vi "Dummy.vi"() -> ()   [LabVIEW 2020]
uses:
  Global 1.vi
panel:
  out "Report Array Header":string[](array[string])
  out "Date (DD/MM/YYYY)":string
  out "SHORT Compensation":string
  out "OPEN Compensation":string
  in  "Calibration Short : Started":bool
  in  "Open Calibration : Started":bool
  in  "Stop Button 2":bool
  out "Current LCR Voltage 2":dbl
  in  "Start Test":bool
  out "Multiplier 2":dbl format="%#_3g"
  out "Test Level value 2":dbl
  in  "Test Comments":string
  in  "Lot Date":timestamp=timestamp(3376684800 s since 1904-01-01) format="%<%x>T"
  in  "Lot Number":string
  in  "Part Number":string
  in  "Request Number":string
  out "TestSigLevel : current time":timestamp
  out "error Mult True":errorcluster
  out "error Mult False":errorcluster
  in  "TestSigLevel : Started":bool
  out "Signal Level : Elapsed time (seconds)":dbl
  in  "OK Button":bool
  in  "Stop Button":bool
  out "Current LCR Voltage":dbl
  out "Multiplier":dbl format="%#_3g"
  out "Test Level Equal":bool
  out "Test Level value":dbl
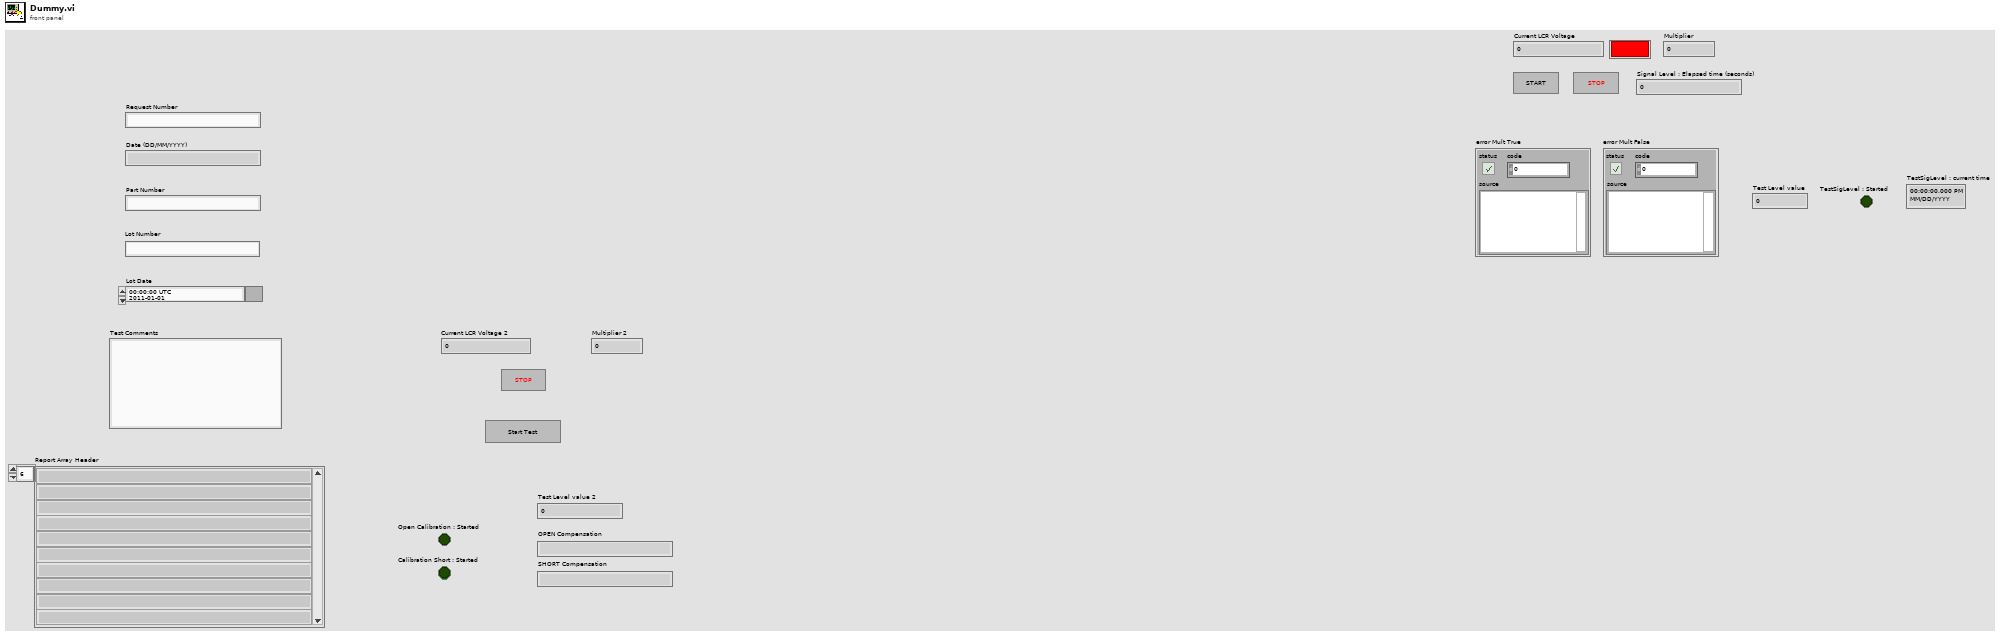
[diagram p1: front panel]
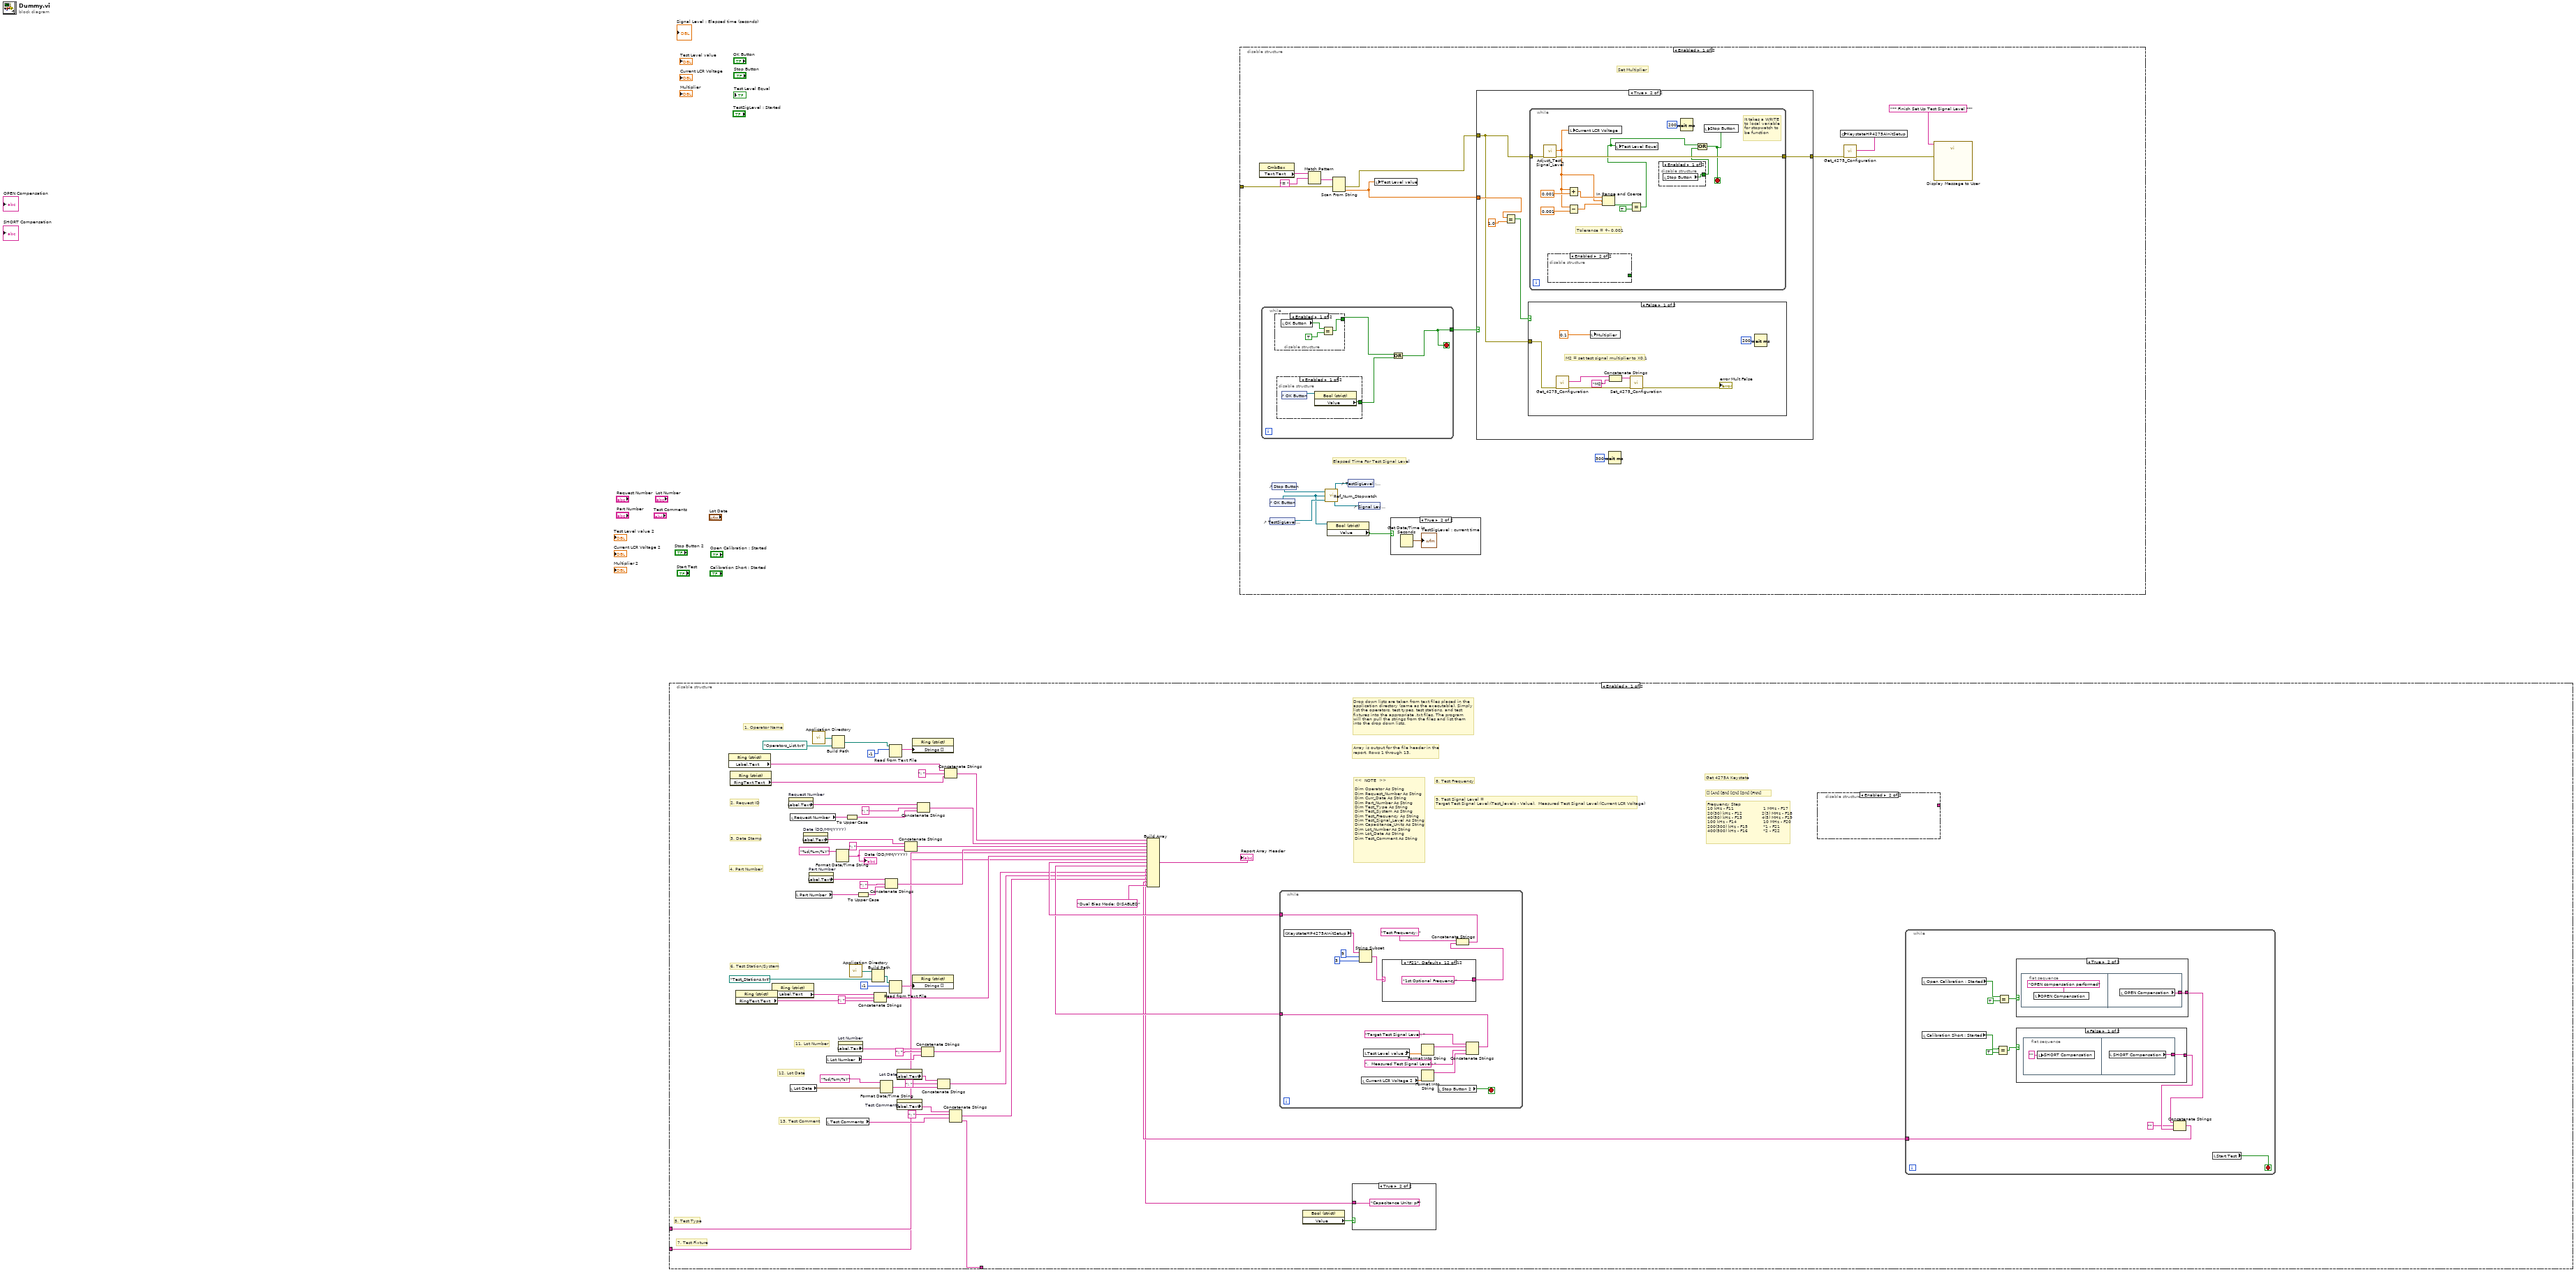
[diagram p0: block diagram]
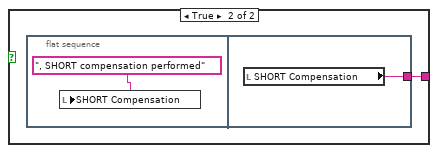
[diagram p2: hidden frame]
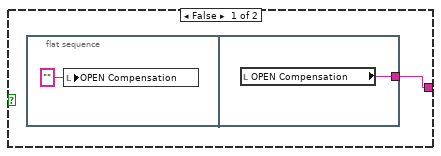
[diagram p3: hidden frame]
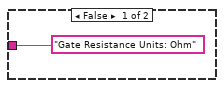
[diagram p4: hidden frame]
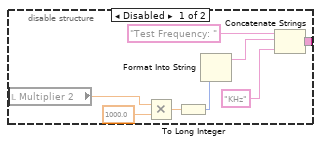
[diagram p5: hidden frame]
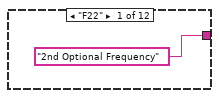
[diagram p6: hidden frame]
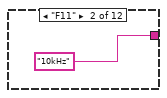
[diagram p7: hidden frame]
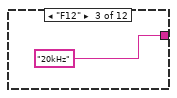
[diagram p8: hidden frame]
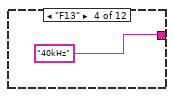
[diagram p9: hidden frame]
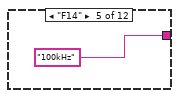
[diagram p10: hidden frame]
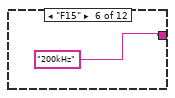
[diagram p11: hidden frame]
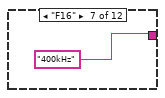
[diagram p12: hidden frame]
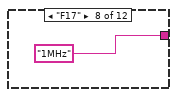
[diagram p13: hidden frame]
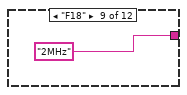
[diagram p14: hidden frame]
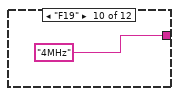
[diagram p15: hidden frame]
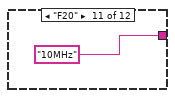
[diagram p16: hidden frame]
diagram:
  n1 = disable-structure shown="Enabled" {
    disable-tunnel: _ -> [w5 _]
    disable-tunnel: _ -> [w4 _]
    disable-tunnel: _ -> [w1 _]
    frame Enabled {
      # "7. Test Fixture"
      # "Frequency Step\n10 kHz - F11                     1 MHz - F17\n20(30) kHz - F12              2(3) MHz - F18\n40(50) kHz - F13              4(5) MHz - F19\n100 kHz - F14                   10 MHz - F20\n200(300) kHz - F15           *1 - F21\n400(500) kHz - F16           *2 - F22"
      # "[] [AN] [BN] [CN] [DN] [FNN]"
      # "Get 4275A Keystate"
      # "8. Test Frequency"
      # "<<  NOTE  >>\n\nDim Operator As String\nDim Request_Number As String\nDim Curr_Date As String\nDim Part_Number As String\nDim Test_Type As String\nDim Test_System As String\nDim Test_Frequency As String\nDim Test_Signal_Level As String\nDim Capacitance_Units As String\nDim Lot_Number As String\nDim Lot_Date As String\nDim Test_Comment As String"
      # "13. Test Comment"
      # "Array is output for the file header in the \nreport. Rows 1 through 13."
      # "Drop down lists are taken from text files placed in the \napplication directory (same as the executable). Simply\nlist the operators, test types, test stations, and test\nfixtures into the appropriate .txt files. The program\nwill then pull the strings from the files and list them\ninto the drop down lists."
      # "12. Lot Date"
      # "11. Lot Number"
      # "9. Test Signal Level = \nTarget Test Signal Level:(Test_levels - Value),  Measured Test Signal Level:(Current LCR Voltage)"
      # "6. Test Station/System"
      # "5. Test Type"
      # "4. Part Number"
      # "3. Date Stamp"
      # "2. Request ID"
      # "1. Operator Name"
      n2 = property on="Property Node" class="Ring (strict)"() -> ("Label.Text"=w29:string)  [unwired: 2 in, 2 out]
      n3 = property on="Property Node" class="Ring (strict)"() -> ("RingText.Text"=w55:string)  [unwired: 2 in, 2 out]
      n4 = property on="Property Node" class="Ring (strict)"() -> ("RingText.Text"=w27:string)  [unwired: 2 in, 2 out]
      n5 = property on="Property Node" class="Ring (strict)"() -> ("Label.Text"=w42:string)  [unwired: 2 in, 2 out]
      n6 = property on="Request Number" class="Str"() -> ("Label.Text"=w54:string)  [unwired: 2 in, 2 out]
      n7 = local read "Lot Date"() -> (w19:timestamp)
      n8 = local read "Request Number"() -> (w31:string)
      n9 = local read "Part Number"() -> (w30:string)
      n10 = property on="Date (DD/MM/YYYY)" class="Str"() -> ("Label.Text"=w51:string)  [unwired: 2 in, 2 out]
      n11 = property on="Part Number" class="Str"() -> ("Label.Text"=w48:string)  [unwired: 2 in, 2 out]
      n12 = call <vilib>:"Application Directory.vi"() -> ("Application Directory"=w37:path)
      n13 = local read "Lot Number"() -> (w25:string)
      n14 = local read "Test Comments"() -> (w21:string)
      n15 = Build Path(base path=w37, name or relative path=path "Operators_List.txt" ("file (use dialog)")) -> (appended path=w35:path)
      n16 = Format Date/Time String(time format string (%c)="%d/%m/%Y") -> (date/time string=w50:string)  [unwired: 2 in]
      "Date (DD/MM/YYYY)" <- w50
      n17 = property on="Lot Number" class="Str"() -> ("Label.Text"=w41:string)  [unwired: 2 in, 2 out]
      n18 = To Upper Case(1:w31) -> (0:w45:string)
      n19 = call <vilib>:"Application Directory.vi"() -> ("Application Directory"=w34:path)
      n20 = To Upper Case(1:w30) -> (0:w46:string)
      n21 = Build Path(base path=w34, name or relative path=path "Test_Stations.txt" ("file (use dialog)")) -> (appended path=w32:path)
      n22 = Concatenate Strings(w42, ": " ("string"), w27) -> (w13:string)
      n23 = Format Date/Time String(time format string (%c)="%d/%m/%Y", seconds (now)=w19) -> (date/time string=w23:string)  [unwired: 1 in]
      n24 = Concatenate Strings(w48, ": " ("string"), w46) -> (w14:string)
      n25 = Read from Text File(file (use dialog)=w35, count=-1) -> (text=w57:string[])  [unwired: 2 in, 3 out]
      n26 = Read from Text File(file (use dialog)=w32, count=-1) -> (text=w43:string[])  [unwired: 2 in, 3 out]
      n27 = property on="Lot Date" class="AbsTime (strict)"() -> ("Label.Text"=w39:string)  [unwired: 2 in, 2 out]
      n28 = property on="Test Comments" class="Str"() -> ("Label.Text"=w38:string)  [unwired: 2 in, 2 out]
      n29 = Concatenate Strings(w51, ": " ("string"), w50) -> (w15:string)
      n30 = property on="Property Node" class="Ring (strict)"("Strings []"=w57) -> ()  [unwired: 2 in, 2 out]
      n31 = property on="Property Node" class="Ring (strict)"("Strings []"=w43) -> ()  [unwired: 2 in, 2 out]
      n32 = Concatenate Strings(w54, ": " ("string"), w45) -> (w16:string)
      n33 = Concatenate Strings(w41, ": " ("string"), w25) -> (w10:string)
      n34 = Concatenate Strings(w39, ": " ("string"), w23) -> (w9:string)
      n35 = Concatenate Strings(w29, ": " ("string"), w55) -> (w17:string)
      n36 = Concatenate Strings(w38, ": " ("string"), w21, w1) -> (w8:string)
      n37 = while {
        tunnel: [w99] -> w11
        tunnel: [w92] -> w12
        stop <- w98 stop-if-true
        n38 = global read "Global 1.vi" "KeystateHP4275AInitSetup"() -> (w91:string)
        n39 = String Subset(string=w91, offset (0)=9, length (rest)=3 ("length (rest)")) -> (substring=w96:string)
        n40 = local read "Current LCR Voltage 2"() -> (w101:dbl)
        n41 = local read "Test Level value 2"() -> (w104:dbl)
        n42 = case shown="\"F21\", Default" w96 {
          tunnel: ["2nd Optional Frequency" "10kHz" "20kHz" "40kHz" "100kHz" "200kHz" "400kHz" "1MHz" "2MHz" "4MHz" "10MHz" "1st Optional Frequency"] -> w93
          frame "F22" {
          }
          frame "F11" {
          }
          frame "F12" {
          }
          frame "F13" {
          }
          frame "F14" {
          }
          frame "F15" {
          }
          frame "F16" {
          }
          frame "F17" {
          }
          frame "F18" {
          }
          frame "F19" {
          }
          frame "F20" {
          }
          frame "F21", Default {
          }
        }
        n43 = Format Into String(w104) -> (resulting string=w103:string)  [unwired: 3 in, 1 out]
        n44 = Format Into String(w101) -> (resulting string=w100:string)  [unwired: 3 in, 1 out]
        n45 = local read "Stop Button 2"() -> (w98:bool)
        n46 = Concatenate Strings("Test Frequency: " ("string"), w93) -> (w92:string)
        n47 = Concatenate Strings("Target Test Signal Level: " ("string"), w103, ",  Measured Test Signal Level: " ("string"), w100) -> (w99:string)
      }
      n48 = property on="Property Node" class="Bool (strict)"() -> ("Value"=w2:bool)  [unwired: 2 in, 2 out]
      n49 = case shown="True" w2 {
        tunnel: ["Gate Resistance Units: Ohm" ("element") "Capacitance Units: pF" ("element")] -> w3
        frame False {
        }
        frame True {
        }
      }
      n50 = disable-structure shown="Enabled" {
        disable-tunnel: [w85 _] -> _
        frame Disabled {
          n51 = local read "Multiplier 2"() -> (w89:dbl)
          n52 = Multiply(x=w89, y=1000.0) -> (x*y=w84:dbl)
          n53 = To Long Integer(number=w84) -> (32bit integer=w83:i32)
          n54 = Format Into String(w83) -> (resulting string=w87:string)  [unwired: 3 in, 1 out]
          n55 = Concatenate Strings("Test Frequency: " ("string"), w87, "KHz" ("string")) -> (w85:string)
        }
        frame Enabled {
        }
      }
      n56 = while {
        tunnel: [w59] -> w6
        stop <- w58 stop-if-true
        n57 = local read "Open Calibration : Started"() -> (w66:bool)
        n58 = local read "Calibration Short : Started"() -> (w64:bool)
        n59 = Equal?(x=w64, y=TRUE) -> (x = y?=w63:bool)
        n60 = Equal?(x=w66, y=TRUE) -> (x = y?=w65:bool)
        n61 = case shown="True" w65 {
          tunnel: [w75 w78] -> w67
          frame False {
            n62 = flat-sequence {
              tunnel: [w77] -> w75
              frame #0 {
                n63 = local write "OPEN Compensation"("" ("OPEN Compensation")) -> ()
              }
              frame #1 {
                n64 = local read "OPEN Compensation"() -> (w77:string)
              }
            }
          }
          frame True {
            n65 = flat-sequence {
              tunnel: [w80] -> w78
              frame #0 {
                n66 = local write "OPEN Compensation"("OPEN compensation performed" ("OPEN Compensation")) -> ()
              }
              frame #1 {
                n67 = local read "OPEN Compensation"() -> (w80:string)
              }
            }
          }
        }
        n68 = case shown="False" w63 {
          tunnel: [w69 w72] -> w68
          frame False {
            n69 = flat-sequence {
              tunnel: [w71] -> w69
              frame #0 {
                n70 = local write "SHORT Compensation"("" ("OPEN Compensation")) -> ()
              }
              frame #1 {
                n71 = local read "SHORT Compensation"() -> (w71:string)
              }
            }
          }
          frame True {
            n72 = flat-sequence {
              tunnel: [w74] -> w72
              frame #0 {
                n73 = local write "SHORT Compensation"(", SHORT compensation performed" ("SHORT Compensation")) -> ()
              }
              frame #1 {
                n74 = local read "SHORT Compensation"() -> (w74:string)
              }
            }
          }
        }
        n75 = Concatenate Strings(w67, "" ("string"), w68) -> (w59:string)
        n76 = local read "Start Test"() -> (w58:bool)
      }
      n77 = Build Array(w17, w16, w15, w14, w5, w13, w4, w12, w11, w3, w10, w9, w8, w6, "Dual Bias Mode: DISABLED" ("element")) -> (→"Report Array Header":string[])
    }
    frame Disabled {
    }
  }
  n78 = disable-structure shown="Enabled" {
    disable-tunnel: _ -> [w121 _]
    frame Enabled {
      # "Elapsed Time For Test Signal Level"
      # "Set Multiplier"
      n79 = property on="Property Node" class="CmbBox"() -> ("Text.Text"=w135:string)  [unwired: 2 in, 2 out]
      n80 = while {
        tunnel: [w136] -> w124
        stop <- w136 stop-if-true
        n81 = disable-structure shown="Enabled" {
          disable-tunnel: [w141 _] -> w138
          frame Enabled {
            n82 = local read "OK Button"() -> (w142:bool)
            n83 = Equal?(x=w142, y=TRUE) -> (x = y?=w141:bool)
          }
          frame Disabled {
          }
        }
        n84 = disable-structure shown="Enabled" {
          disable-tunnel: [w139 _] -> w137
          frame Enabled {
            n85 = control-ref of="OK Button"() -> (w140:refnum<vi>)
            n86 = property class="Bool (strict)"(reference=w140) -> ("Value"=w139:bool)  [unwired: 1 in, 2 out]
          }
          frame Disabled {
          }
        }
        n87 = Or(x=w138, y=w137) -> (x .or. y?=w136:bool)
      }
      n88 = control-ref of="OK Button"() -> (w126:refnum<vi>)
      n89 = control-ref of="TestSigLevel : Started"() -> (w128:refnum<vi>)
      n90 = control-ref of="Stop Button"() -> (w129:refnum<vi>)
      n91 = Match Pattern(string=w135, regular expression="= ") -> (after substring=w133:string)  [unwired: 1 in, 3 out]
      n92 = property class="Bool (strict)"(reference=w126) -> ("Value"=w125:bool)  [unwired: 1 in, 2 out]
      n93 = Scan From String(input string=w133, error in=w121) -> (error out=w122:errorcluster, output 1=w131:dbl)  [unwired: 3 in, 2 out]
      n94 = control-ref of="TestSigLevel : current time"() -> (w127:refnum<vi>)
      n95 = control-ref of="Signal Level : Elapsed time (seconds)"() -> (w130:refnum<vi>)
      n96 = call "Ref_Num_Stopwatch.vi"("Elapsed time (seconds)"=w130, "start time"=w127, "Started"=w128, "OK Button"=w126, "stop"=w129) -> ()  [unwired: 1 in]
      n97 = local write "Test Level value"(w131) -> ()
      n98 = case shown="True" w125 {
        frame False {
        }
        frame True {
          n99 = Get Date/Time In Seconds() -> (seconds since 1Jan1904=→"TestSigLevel : current time":timestamp)
        }
      }
      n100 = case shown="True" w124 {
        tunnel: w122 -> [w144 w146]
        tunnel: w131 -> [_ w147]
        tunnel: [w144 w145] -> w120
        frame False {
        }
        frame True {
          n101 = Equal?(x=w147, y=1.0) -> (x = y?=w149:bool)
          n102 = case shown="False" w149 {
            tunnel: w146 -> [w152 w158]
            frame False {
              # "M2 = set test signal multiplier to X0.1"
              n103 = call "Get_4275_Configuration.vi"("error in"=w152) -> ("error out"=w151:errorcluster, "Keystate"=w155:string)  [unwired: 9 in]
              n104 = local write "Multiplier"(0.1) -> ()
              n105 = Concatenate Strings(w155, "M2" ("string")) -> (w154:string)
              n106 = call "Set_4275_Configuration.vi"("error in"=w151, "Keystate"=w154) -> ("error out"=→"error Mult False":errorcluster)  [unwired: 9 in]
              n107 = Wait (ms)(milliseconds to wait=u32 200) -> ()  [unwired: 1 out]
            }
            frame True {
              # "M3 = set test signal multiplier to X1"
              n108 = call "Get_4275_Configuration.vi"("error in"=w158) -> ("error out"=w160:errorcluster, "Keystate"=w164:string)  [unwired: 9 in]
              n109 = local write "Multiplier"(1.0 ("Multiplier")) -> ()
              n110 = Concatenate Strings(w164, "M3" ("string")) -> (w162:string)
              n111 = call "Set_4275_Configuration.vi"("error in"=w160, "Keystate"=w162) -> ("error out"=→"error Mult True":errorcluster)  [unwired: 9 in]
              n112 = Wait (ms)(milliseconds to wait=u32 200) -> ()  [unwired: 1 out]
            }
          }
          n113 = while {
            tunnel: w146 -> [w178]
            tunnel: [w177] -> w145
            stop <- w174 stop-if-true
            # "Tolerance = +- 0.001"
            # "It takes a WRITE\nto local variable\nfor stopwatch to \nbe function"
            n114 = call "Adjust_Test_Signal_Level.vi"("error in"=w178) -> ("error out"=w177:errorcluster, "OscVoltage"=w169:dbl)  [unwired: 9 in]
            n115 = disable-structure shown="Enabled" {
              disable-tunnel: [w179 _] -> _
              frame Disabled {
                n116 = control-ref of="Stop Button"() -> (w180:refnum<vi>)
                n117 = property class="Bool (strict)"(reference=w180) -> ("Value"=w179:bool)  [unwired: 1 in, 2 out]
              }
              frame Enabled {
              }
            }
            n118 = Add(x=w169, y=0.001) -> (x+y=w171:dbl)
            n119 = Subtract(x=w169, y=0.001) -> (x-y=w170:dbl)
            n120 = local write "Current LCR Voltage"(w169) -> ()
            n121 = In Range and Coerce(upper limit=w171, x=w169, lower limit=w170) -> (In Range?=w168:bool)  [unwired: 1 out]
            n122 = Equal?(x=w168, y=TRUE) -> (x = y?=w166:bool)
            n123 = local write "Test Level Equal"(w166) -> ()
            n124 = disable-structure shown="Enabled" {
              disable-tunnel: [w181 _] -> w175
              frame Enabled {
                n125 = local read "Stop Button"() -> (w181:bool)
              }
              frame Disabled {
              }
            }
            n126 = Wait (ms)(milliseconds to wait=u32 200) -> ()  [unwired: 1 out]
            n127 = Or(x=w166, y=w175) -> (x .or. y?=w174:bool)
            n128 = local write "Stop Button"(w174) -> ()
          }
        }
      }
      n129 = Wait (ms)(milliseconds to wait=u32 300) -> ()  [unwired: 1 out]
      n130 = call "Get_4275_Configuration.vi"("error in"=w120) -> ("error out"=w119:errorcluster, "Keystate"=w118:string)  [unwired: 9 in]
      n131 = global write "Global 1.vi" "KeystateHP4275AInitSetup"(w118) -> ()
      n132 = call "Display Message to User"("error in (no error)"=w119, "Message"="** Finish Set Up Test Signal Level **" ("message")) -> ()  [unwired: 8 in, 2 out]
    }
    frame Disabled {
    }
  }
